vi "Make Permutations.vi"(11 "String":string) -> (3 "Array":string[](array[string]))   [LabVIEW 2020]
uses:
  a49ac8f5-ccab-4f45-af8e-d0127a0646c9.vi
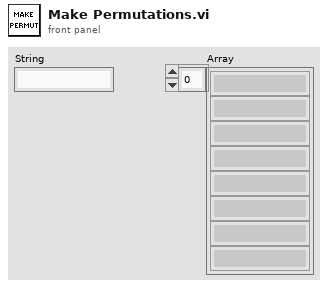
[diagram p1: front panel]
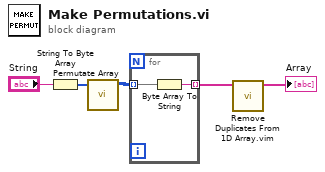
[diagram p0: block diagram]
diagram:
  n1 = String To Byte Array(string="String") -> (unsigned byte array=w1:u8[])
  n2 = call "Permutate Array.vi"("unsigned byte array in"=w1) -> ("unsigned byte array out"=w4:u8[][])  [unwired: 10 in]
  n3 = for {
    tunnel: w4 -> [w7] mode=indexing
    tunnel: [w6] -> w3 mode=indexing
    n4 = Byte Array To String(unsigned byte array=w7) -> (string=w6:string)
  }
  n5 = call "Remove Duplicates From 1D Array.vim"("array"=w3) -> ("array with duplicates removed"=→"Array":string[])  [unwired: 10 in]
